vi "(SubVI)DW7800.vi"() -> ()   [LabVIEW 2020]
uses:
  <vilib>/Utility/miscctls.llb/LVPointTypeDef.ctl
  Libraries/Haptic IC Class/Haptic IC/Haptic IC.lvclass/Haptic IC.ctl
  Waveform Editor/Controls/(Ctrl)Waveform Editor_Update Sampling Rate Value.ctl
  Libraries/Haptic IC Class/Haptic IC/Accessors/Write freq ref.vi
  Libraries/Haptic IC Class/Haptic IC/Accessors/Write voltage range ref.vi
  Variables/(Var)System Variables.vi
  I2C/Instance VIs/(SubVI)I2C_8Bit-8Bit_Read_Single.vi
  I2C/Instance VIs/(SubVI)I2C_8Bit-8Bit_Write_Single.vi
  Libraries/Haptic IC Class/Haptic IC/Haptic IC.lvclass
panel:
  in  "Stop":bool
  in  "탭 컨트롤":enum32{"Common"}(tab)
  out "Status_Result":string
  out "Packet Size":u8(ring) items=["0 byte", "1 byte", "2 byte", "3 byte", "4 byte", "5 byte", "6 byte", "7 byte", "8 byte", "9 byte", "10 byte", "11 byte", "12 byte", "13 byte", "14 byte", "15 byte", "16 byte", "17 byte", "18 byte", "19 byte", "20 byte", "21 byte", "22 byte", "23 byte", "24 byte", "25 byte", "26 byte", "27 byte", "28 byte", "29 byte", "30 byte", "31 byte", "32 byte", "33 byte", "34 byte", "35 byte", "36 byte", "37 byte", "38 byte", "39 byte", "40 byte", "reserved", "reserved", "reserved", "reserved", "reserved", "reserved", "reserved", "reserved", "reserved", "reserved", "reserved", "reserved", "reserved", "reserved", "reserved", "reserved", "reserved", "reserved", "reserved", "reserved", "reserved", "reserved", "reserved", "reserved", "reserved", "reserved", "over 40 byte"]
  in  "HW Reset Disble":bool caption="HW Reset Disable"
  in  "LDO Level":u8(ring) caption="LDO" items=["1.2V", "1.4V", "1.6V", "1.8V", "2.0V", "2.2V", "2.4V", "2.6V", "2.8V", "3.0V", "3.2V", "3.4V", "3.6V", "reserved", "reserved", "reserved"]
  in  "Timing Set_HTIME":enum8{"0ms", "5ms", "10ms", "20ms"}(ring)=enum."5ms" caption="Hold Time"
  in  "Timing Set_FREQ":enum8{"8kHz", "4kHz", "2kHz", "1kHz"}(ring) caption="Freq."
  out "FIFO Fullness":T1(ring)
  in  "SW Reset":bool
  in  "Read All":bool
  # "STATUS"
  # "FIFO FULLNESS"
  # "SW RESET"
  # "TIMING SET"
  # "LDO LEVEL"
  # "HW RESET DISABLE"
  # "PACKET SIZE"
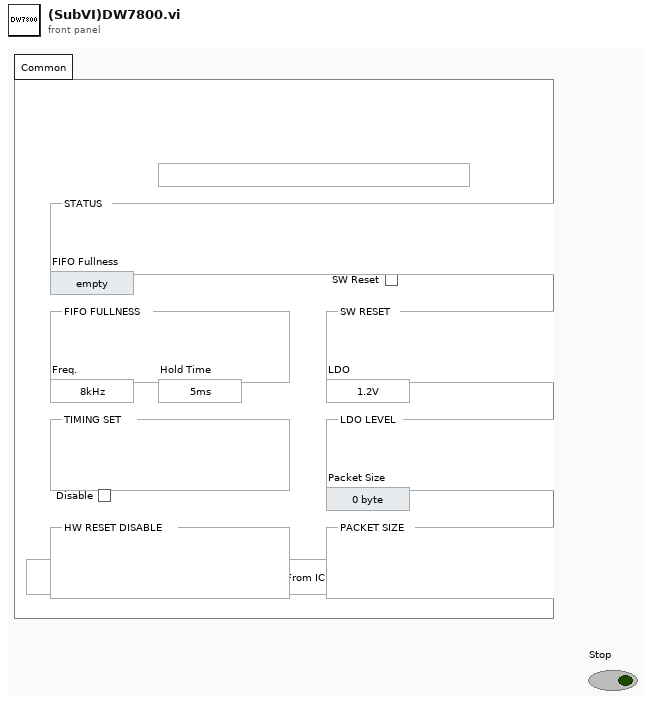
[diagram p1: front panel]
types:
  T1 = enum8{"empty", "1", "2", "3", "4", "5", "6", "7", "8", "9", "10", "11", "12", "13", "14", "15", "16", "17", "18", "19", "20", "21", "22", "23", "24", "25", "26", "27", "28", "29", "30", "31", "32", "33", "34", "35", "36", "37", "38", "39", "40", "41", "42", "43", "44", "45", "46", "47", "48", "49", "50", "51", "52", "53", "54", "55", "56", "57", "58", "59", "60", "61", "62", "63", "64", "65", "66", "67", "68", "69", "70", "71", "72", "73", "74", "75", "76", "77", "78", "79", "80", "81", "82", "83", "84", "85", "86", "87", "88", "89", "90", "91", "92", "93", "94", "95", "96", "97", "98", "99", "100", "101", "102", "103", "104", "105", "106", "107", "108", "109", "110", "111", "112", "113", "114", "115", "116", "117", "118", "119", "120", "121", "122", "123", "124", "125", "126", "127", "full"}
  T2 = typedef "LVPointTypeDef.ctl" = cluster{"Horizontal":i16, "Vertical":i16}
  T3 = typedef "(Ctrl)Waveform Editor_Update Sampling Rate Value.ctl" = enum16{"Init", "Update"}
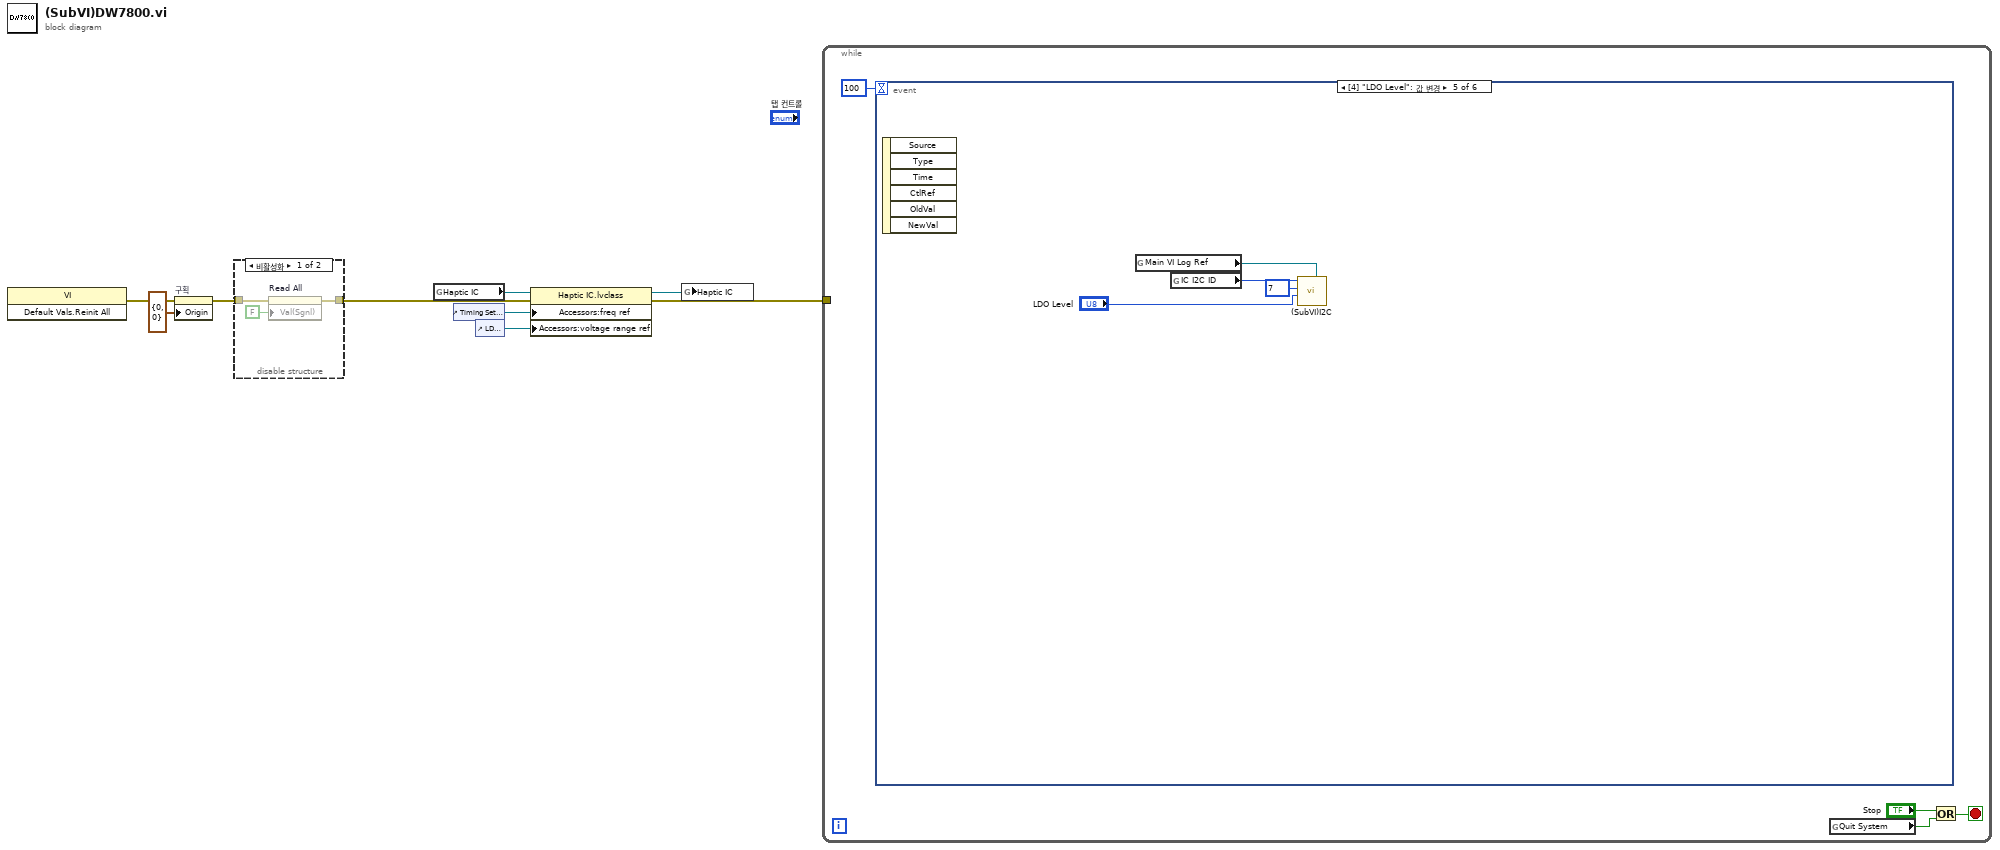
[diagram p0: block diagram]
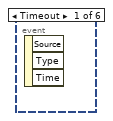
[diagram p3: hidden frame]
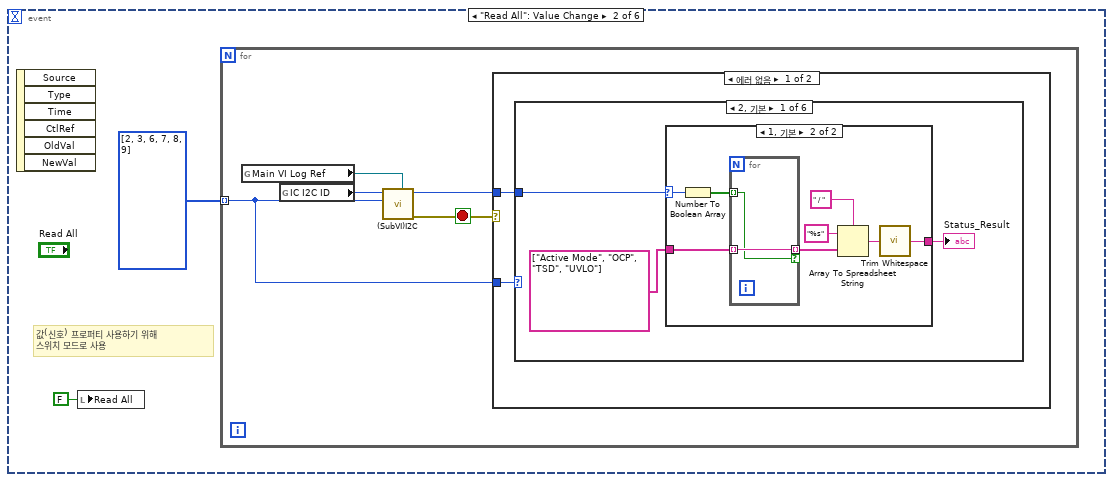
[diagram p4: hidden frame]
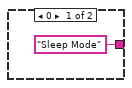
[diagram p5: hidden frame]
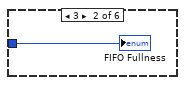
[diagram p6: hidden frame]
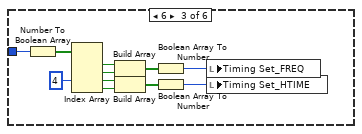
[diagram p7: hidden frame]
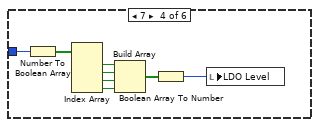
[diagram p8: hidden frame]
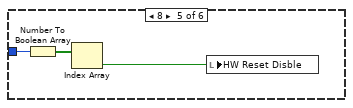
[diagram p9: hidden frame]
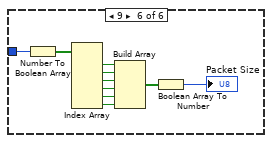
[diagram p10: hidden frame]
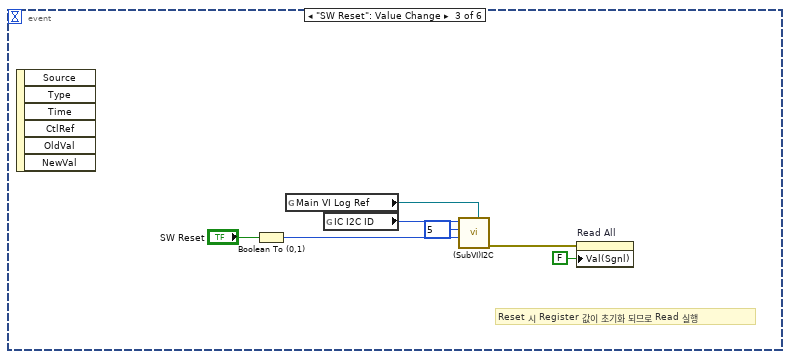
[diagram p12: hidden frame]
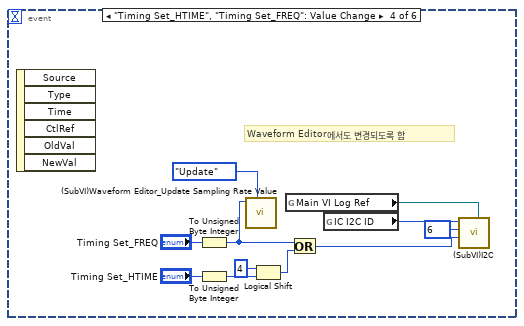
[diagram p13: hidden frame]
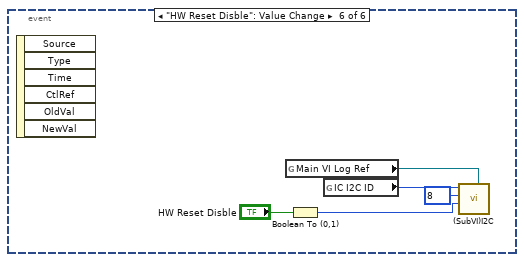
[diagram p14: hidden frame]
diagram:
  n1 = invoke class="VI" method="Default Vals.Reinit All"() -> (error out=w9:errorcluster)  [unwired: 3 in, 2 out]
  n2 = property on="구획" class="Pane"(error in=w9, "Origin"=T2 {"Horizontal"=0, "Vertical"=0} ("원점")) -> (error out=w7:errorcluster)  [unwired: 1 in, 1 out]
  n3 = disable-structure shown="비활성화" {
    disable-tunnel: w7 -> [w12 w13]
    disable-tunnel: [w11 w13] -> w5
    frame Disabled {
      n4 = property on="Read All" class="Bool (엄격한)"(error in=w12, "Val(Sgnl)"=FALSE ("값(신호)")) -> (error out=w11:errorcluster)  [unwired: 1 in, 1 out]
    }
    frame Enabled {
    }
  }
  n5 = global read "(Var)System Variables.vi" "Haptic IC"() -> (w6:refnum<class "Haptic IC.lvclass">)
  n6 = control-ref of="Timing Set_FREQ"() -> (w3:refnum<vi>)
  n7 = control-ref of="LDO Level"() -> (w2:refnum<vi>)
  n8 = property class="Haptic IC.lvclass"(reference=w6, error in=w5, "Accessors:freq ref"=w3, "Accessors:voltage range ref"=w2) -> (reference out=w1:refnum<class "Haptic IC.lvclass">, error out=w4:errorcluster)
  n9 = global write "(Var)System Variables.vi" "Haptic IC"(w1) -> ()
  n10 = while {
    tunnel: w4 -> [_]
    stop <- w15 stop-if-true
    n11 = event shown="[4] \"LDO Level\": 값 변경" {
      selector: _ -> [_ _ _ _ _ _]
      dyn-events: _ -> [_ _ _ _ _ _]
      timeout: 100 -> [_ _ _ _ _ _]
      event Timeout {
        n12 = event-data() -> ()  [unwired: 1 in, 3 out]
      }
      event "Read All": Value Change {
        # "값(신호) 프로퍼티 사용하기 위해\n스위치 모드로 사용"
        n13 = event-data() -> ()  [unwired: 1 in, 6 out]
        n14 = local write "Read All"(FALSE ("Read All")) -> ()
        n15 = for {
          tunnel: u8[] [2, 3, 6, 7, 8, 9] -> [w21] mode=indexing
          stop <- w20 stop-if-true
          n16 = global read "(Var)System Variables.vi" "Main VI Log Ref"() -> (w23:refnum<vi>)
          n17 = global read "(Var)System Variables.vi" "IC I2C ID"() -> (w24:u8)
          n18 = call-poly "(SubVI)I2C.vi"("Log Ref"=w23, "Address"=w21, "ID"=w24) -> ("error out"=w20:errorcluster, "Read Data"=w22:u8)  [unwired: 6 in, 1 out]
          n19 = case shown="에러 없음" w20 {
            tunnel: w22 -> [w26 _]
            tunnel: w21 -> [w25 _]
            frame No Error {
              n20 = case shown="2, 기본" w25 {
                tunnel: w26 -> [w29 w41 w52 w60 w63 w73]
                frame 2, Default {
                  n21 = case shown="1, 기본" w29 {
                    selector: w29 -> [_ w38]
                    tunnel: string[] ["Active Mode", "OCP", "TSD", "UVLO"] -> [_ w36]
                    tunnel: ["Sleep Mode" ("trimmed string") w31] -> w28
                    frame 0 {
                    }
                    frame 1, Default {
                      n22 = Number To Boolean Array(number=w38) -> (Boolean array=w37:bool[])
                      n23 = for {
                        tunnel: w37 -> [w39] mode=indexing
                        tunnel: w36 -> [w40] mode=indexing
                        tunnel: [w40] -> w35 mode=indexing if=w39
                      }
                      n24 = Array To Spreadsheet String(delimiter (Tab)=" / " ("구분 문자 (탭)"), array=w35, 3:"%s" ("포맷 문자열")) -> (spreadsheet string=w32:string)
                      n25 = call <vilib>:"Trim Whitespace.vi"("string"=w32) -> ("trimmed string"=w31:string)  [unwired: 1 in]
                    }
                  }
                  "Status_Result" <- w28
                }
                frame 3 {
                  "FIFO Fullness" <- w41
                }
                frame 6 {
                  n26 = Number To Boolean Array(number=w52) -> (Boolean array=w51:bool[])
                  n27 = Index Array(array=w51, index #3=4 ("인덱스")) -> (element #1=w49:bool, element #2=w48:bool, element #3=w47:bool, element #4=w46:bool)  [unwired: 3 in]
                  n28 = Build Array(w49, w48) -> (w45:bool[])
                  n29 = Build Array(w47, w46) -> (w44:bool[])
                  n30 = Boolean Array To Number ("불리언 배열을 숫자로")(Boolean array=w45) -> (number=w43:u8)
                  n31 = Boolean Array To Number ("불리언 배열을 숫자로")(Boolean array=w44) -> (number=w42:u8)
                  n32 = local write "Timing Set_FREQ"(w43) -> ()
                  n33 = local write "Timing Set_HTIME"(w42) -> ()
                }
                frame 7 {
                  n34 = Number To Boolean Array(number=w60) -> (Boolean array=w59:bool[])
                  n35 = Index Array(array=w59) -> (element #1=w58:bool, element #2=w57:bool, element #3=w54:bool, element #4=w53:bool)  [unwired: 4 in]
                  n36 = Build Array(w58, w57, w54, w53) -> (w56:bool[])
                  n37 = Boolean Array To Number ("불리언 배열을 숫자로")(Boolean array=w56) -> (number=w55:u8)
                  n38 = local write "LDO Level"(w55) -> ()
                }
                frame 8 {
                  n39 = Number To Boolean Array(number=w63) -> (Boolean array=w62:bool[])
                  n40 = Index Array(array=w62) -> (element=w61:bool)  [unwired: 1 in]
                  n41 = local write "HW Reset Disble"(w61) -> ()
                }
                frame 9 {
                  n42 = Number To Boolean Array(number=w73) -> (Boolean array=w72:bool[])
                  n43 = Index Array(array=w72) -> (element #1=w71:bool, element #2=w70:bool, element #3=w68:bool, element #4=w67:bool, element #5=w66:bool, element #6=w65:bool)  [unwired: 6 in]
                  n44 = Build Array(w71, w70, w68, w67, w66, w65) -> (w69:bool[])
                  n45 = Boolean Array To Number ("불리언 배열을 숫자로")(Boolean array=w69) -> (number=→"Packet Size":u8)
                }
              }
            }
            frame Error {
            }
          }
        }
      }
      event "SW Reset": Value Change {
        # "Reset 시 Register 값이 초기화 되므로 Read 실행"
        n46 = event-data() -> ()  [unwired: 1 in, 6 out]
        n47 = Boolean To (0,1)(Boolean="SW Reset") -> (0, 1=w78:i16)
        n48 = global read "(Var)System Variables.vi" "Main VI Log Ref"() -> (w79:refnum<vi>)
        n49 = global read "(Var)System Variables.vi" "IC I2C ID"() -> (w80:u8)
        n50 = call-poly "(SubVI)I2C.vi"("Log Ref"=w79, "Data to Write"=w78, "Address"=u8 5, "ID"=w80) -> ("error out"=w75:errorcluster)  [unwired: 6 in, 1 out]
        n51 = property on="Read All" class="Bool (엄격한)"(error in=w75, "Val(Sgnl)"=FALSE ("값(신호)")) -> ()  [unwired: 1 in, 2 out]
      }
      event "Timing Set_HTIME", "Timing Set_FREQ": Value Change {
        # "Waveform Editor에서도 변경되도록 함"
        n52 = event-data() -> ()  [unwired: 1 in, 6 out]
        n53 = To Unsigned Byte Integer(number="Timing Set_FREQ") -> (unsigned 8bit integer=w81:u8)
        n54 = To Unsigned Byte Integer(number="Timing Set_HTIME") -> (unsigned 8bit integer=w84:u8)
        n55 = call "(SubVI)Waveform Editor_Update Sampling Rate Value.vi"("Action"=(Ctrl)Waveform_Editor_Update_Sampling_Rate_Value."Update", "Value"=w81) -> ()  [unwired: 9 in, 1 out]
        n56 = Logical Shift(y=i16 4, x=w84) -> (x << y=w86:u8)
        n57 = global read "(Var)System Variables.vi" "Main VI Log Ref"() -> (w90:refnum<vi>)
        n58 = Or(x=w81, y=w86) -> (x .or. y?=w85:u8)
        n59 = global read "(Var)System Variables.vi" "IC I2C ID"() -> (w91:u8)
        n60 = call-poly "(SubVI)I2C.vi"("Log Ref"=w90, "Data to Write"=w85, "Address"=u8 6, "ID"=w91) -> ()  [unwired: 6 in, 2 out]
      }
      event "LDO Level": Value Change {
        n61 = event-data() -> ()  [unwired: 1 in, 6 out]
        n62 = global read "(Var)System Variables.vi" "Main VI Log Ref"() -> (w94:refnum<vi>)
        n63 = global read "(Var)System Variables.vi" "IC I2C ID"() -> (w95:u8)
        n64 = call-poly "(SubVI)I2C.vi"("Log Ref"=w94, "Data to Write"="LDO Level", "Address"=u8 7, "ID"=w95) -> ()  [unwired: 6 in, 2 out]
      }
      event "HW Reset Disble": Value Change {
        n65 = event-data() -> ()  [unwired: 1 in, 6 out]
        n66 = global read "(Var)System Variables.vi" "Main VI Log Ref"() -> (w99:refnum<vi>)
        n67 = Boolean To (0,1)(Boolean="HW Reset Disble") -> (0, 1=w97:i16)
        n68 = global read "(Var)System Variables.vi" "IC I2C ID"() -> (w100:u8)
        n69 = call-poly "(SubVI)I2C.vi"("Log Ref"=w99, "Data to Write"=w97, "Address"=u8 8, "ID"=w100) -> ()  [unwired: 6 in, 2 out]
      }
    }
    n70 = global read "(Var)System Variables.vi" "Quit System"() -> (w16:bool)
    n71 = Or(x="Stop", y=w16) -> (x .or. y?=w15:bool)
  }
